vi "3_OutQueue.vi"(8 "error in (no error)":errorcluster caption="错误输入（无错误）", 10 "QueueName":T2, 11 "Queue In":refnum<queue>[](array[refnum])) -> (0 "error out":errorcluster caption="错误输出", 2 "Data":cluster{"Cmd":T1, "Data":variant}, 3 "QueueOut":refnum<queue>[](array[refnum]))   [LabVIEW 2017]
uses:
  Ctrls/QueueDataForm.ctl
  Ctrls/QueueName.ctl
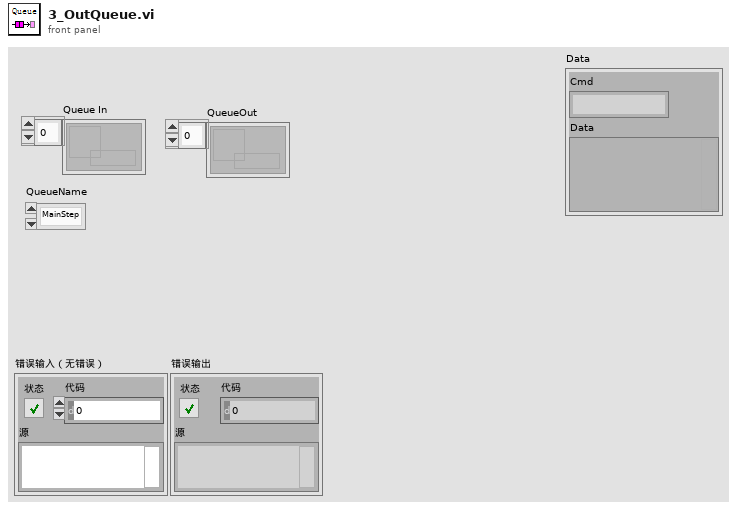
[diagram p1: front panel]
types:
  T1 = typedef "QueueDataForm.ctl" = string
  T2 = typedef "QueueName.ctl" = enum16{"MainStep", "AutoRun", "胶高"}
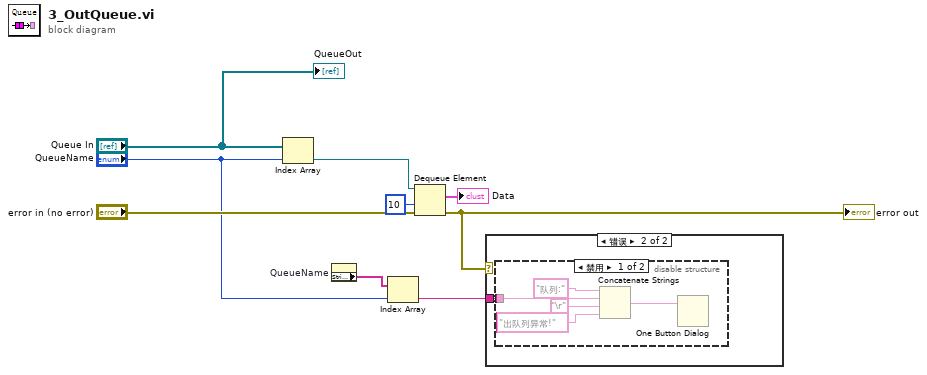
[diagram p0: block diagram]
diagram:
  n1 = Index Array(array="Queue In", index="QueueName") -> (element=w8:refnum<queue>)
  n2 = property on="QueueName" class="Enum (strict)"() -> ("Strings []"=w4:string[])  [unwired: 2 in, 2 out]
  n3 = Index Array(array=w4, index="QueueName") -> (element=w2:string)
  n4 = Dequeue Element(queue=w8, timeout in ms (-1)=10 ("超时毫秒(-1)"), error in (no error)="error in (no error)") -> (element=→"Data":cluster{"Cmd":T1, "Data":variant}, error out=w5:errorcluster)  [unwired: 2 out]
  "error out" <- w5
  n5 = case shown="错误" w5 {
    tunnel: w2 -> [_ w10]
    frame No Error {
    }
    frame Error {
      n6 = disable-structure shown="禁用" {
        disable-tunnel: w10 -> [w14 _]
        frame Disabled {
          n7 = Concatenate Strings("队列:", w14, "\r", "出队列异常!" ("字符串")) -> (w11:string)
          n8 = One Button Dialog(message=w11) -> ()  [unwired: 1 in, 1 out]
        }
        frame Enabled {
        }
      }
    }
  }
  "QueueOut" <- "Queue In"
